vi "FTP自动升级更新main.vi"() -> ()   [LabVIEW 2016, in "自动更新.lvlib"]
uses:
  <vilib>/FTP/NI_FTP.lvlib
panel:
  out "有新版本":bool
  out "最新版本获取进度":u8(slide) scale=0.0..100.0
  # "版本获取中，请稍后！"
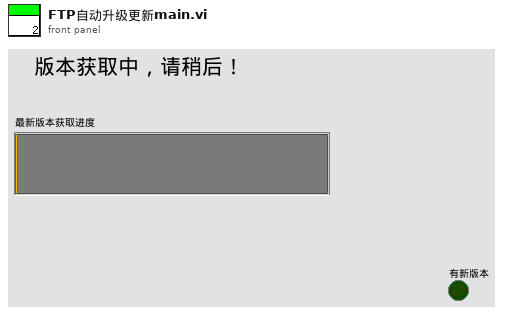
[diagram p1: front panel]
types:
  T1 = enum16{"get version information", "get success", "contact", "over"}
  T2 = cluster{"网络灯":bool, "接收中":bool, "已接收百分比":u8, "接收成功次数":dbl, "当前步骤":enum16{"init", "receivehead", "receivecontent", "receivesuccess", "over"}, "文件名":string, "error out":errorcluster}
  T3 = enum16{"open", "replace", "create", "open or create", "replace or create", "replace or create with confirmation"}
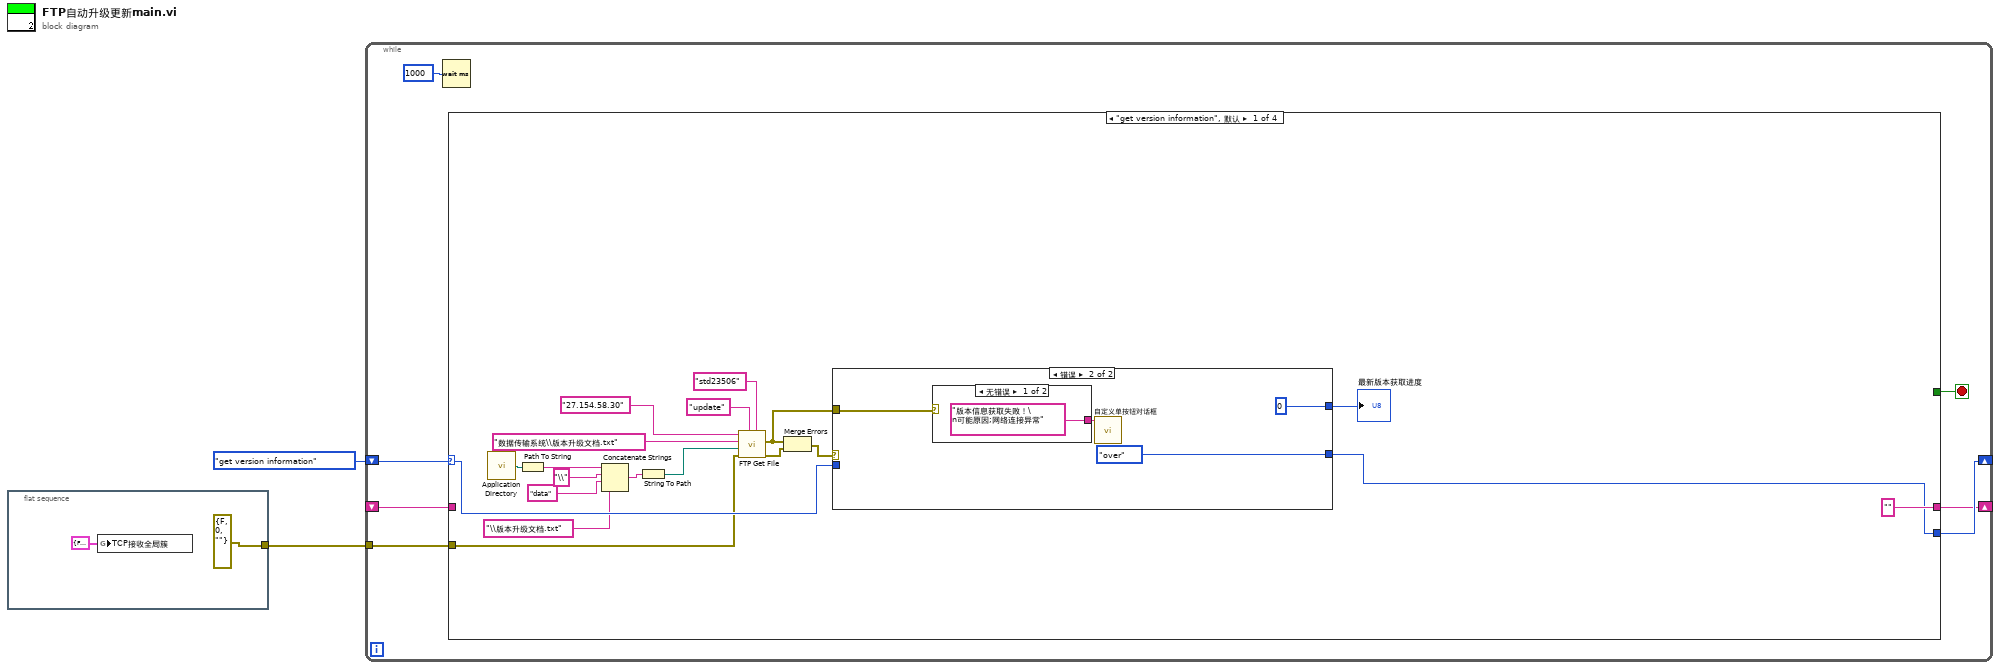
[diagram p0: block diagram]
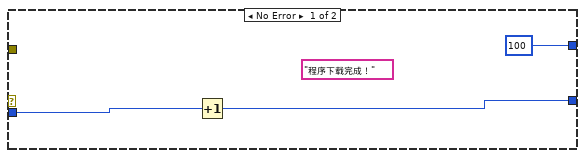
[diagram p2: hidden frame]
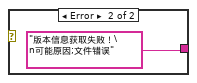
[diagram p3: hidden frame]
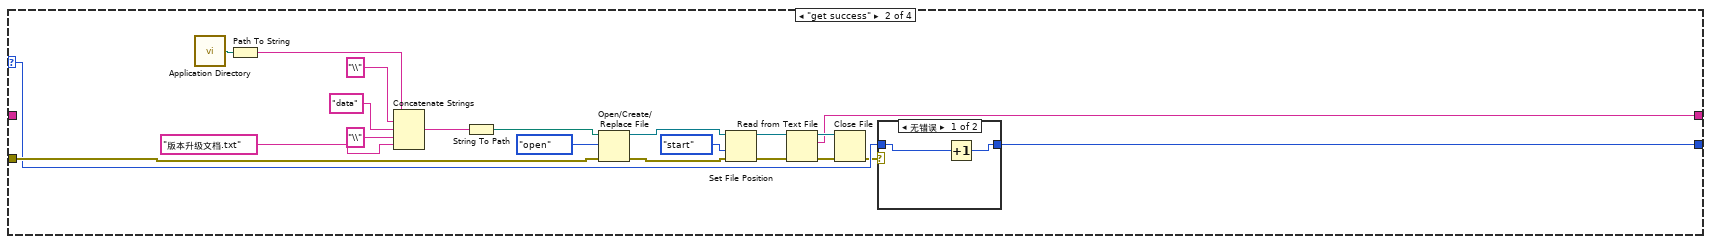
[diagram p4: hidden frame]
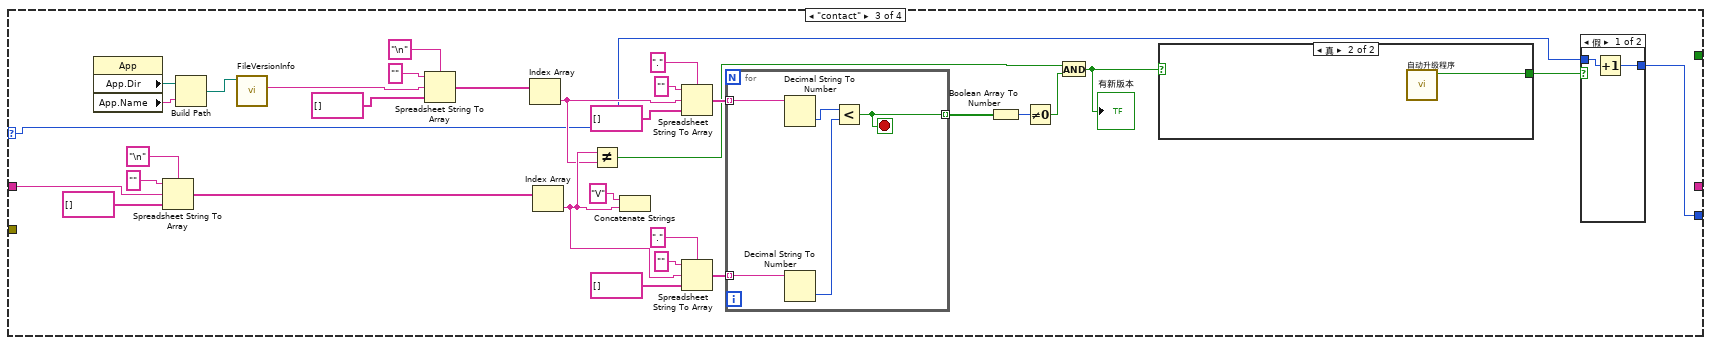
[diagram p6: hidden frame]
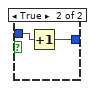
[diagram p7: hidden frame]
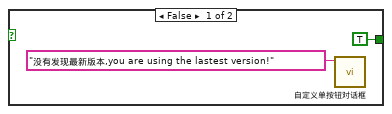
[diagram p8: hidden frame]
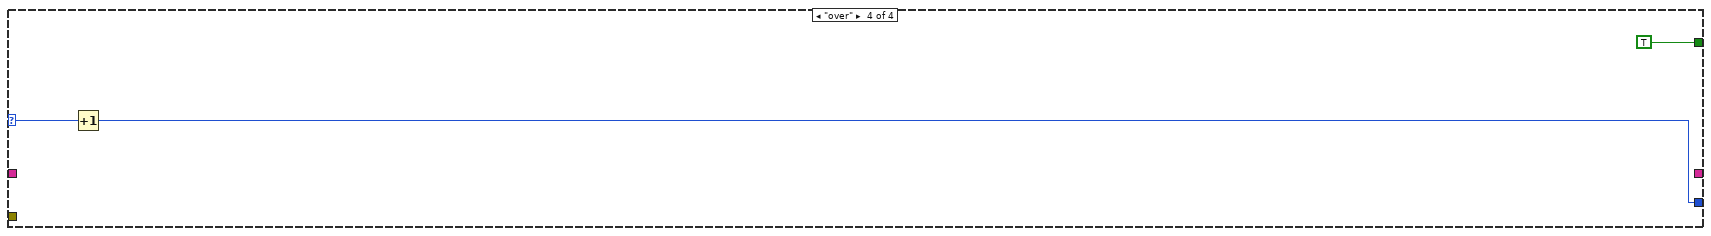
[diagram p9: hidden frame]
diagram:
  n1 = flat-sequence {
    tunnel: [errorcluster {"status"=FALSE, "code"=0, "source"=""} ("错误常量")] -> w1
    frame #0 {
      n2 = global write "全局变量1.vi" "TCP接收全局簇"(T2 {"网络灯"=FALSE, "接收中"=FALSE, "已接收百分比"=0, "接收成功次数"=0.0, "当前步骤"=enum."init", "文件名"="", "error out"={"status"=FALSE, "code"=0, "source"=""}} ("TCP接收全局簇")) -> ()
    }
  }
  n3 = while {
    shift-right: [w9] -> _
    shift-left: T1."get version information" -> [w10]
    tunnel: w1 -> [w8]
    shift-right: [w7] -> _
    shift-left: _ -> [w6]
    stop <- w5 stop-if-true
    n4 = Wait (ms)(milliseconds to wait=u32 1000 ("等待时间（毫秒）")) -> ()  [unwired: 1 out]
    n5 = case shown="\"get version information\", 默认" w10 {
      selector: w10 -> [w15 w47 w69 w109]
      tunnel: [w14 w46 w68 w108] -> w9
      tunnel: w8 -> [w13 w48 _ _]
      tunnel: ["" w40 _ _] -> w7
      tunnel: w6 -> [_ _ w72 _]
      tunnel: [_ _ _ TRUE] -> w5
      frame "get version information", Default {
        n6 = call <vilib>:"Application Directory.vi"() -> ("Application Directory"=w24:path)
        n7 = Path To String(path=w24) -> (string=w27:string)
        n8 = Concatenate Strings(w27, "\\" ("字符串"), "data" ("字符串"), "\\版本升级文档.txt") -> (w23:string)
        n9 = String To Path(string=w23) -> (path=w22:path)
        n10 = call <vilib>:"FTP Get File.vi"("password"="std23506", "user"="update", "error in (no error)"=w13, "local path"=w22, "remote path"="数据传输系统\\版本升级文档.txt", "host"="27.154.58.30") -> ("error out"=w19:errorcluster, "file error"=w17:errorcluster)  [unwired: 4 in]
        n11 = Merge Errors(w17, w19) -> (w18:errorcluster)
        n12 = case shown="错误" w18 {
          tunnel: w17 -> [_ w36]
          tunnel: [u8 100 ("y") u8 0 ("y")] -> w16
          tunnel: [w32 T1."over"] -> w14
          tunnel: w15 -> [w31 _]
          frame No Error {
            (unwired) "程序下载完成！"
            n13 = Increment(x=w31) -> (x+1=w32:T1)
          }
          frame Error {
            n14 = case shown="无错误" w36 {
              tunnel: ["版本信息获取失败！\n可能原因;网络连接异常" "版本信息获取失败！\n可能原因;文件错误"] -> w37
              frame No Error {
              }
              frame Error {
              }
            }
            n15 = call "自定义单按钮对话框.vi"("消息"=w37) -> ()  [unwired: 11 in]
          }
        }
        "最新版本获取进度" <- w16
      }
      frame "get success" {
        n16 = call <vilib>:"Application Directory.vi"() -> ("Application Directory"=w53:path)
        n17 = Path To String(path=w53) -> (string=w56:string)
        n18 = Concatenate Strings(w56, "\\" ("字符串"), "data" ("字符串"), "\\" ("字符串"), "版本升级文档.txt" ("字符串")) -> (w50:string)
        n19 = String To Path(string=w50) -> (path=w49:path)
        n20 = Open/Create/Replace File(file path (use dialog)=w49, error in=w48, operation (0:open)=T3."open" ("操作(0:open)")) -> (refnum out=w59:refnum<file>, error out=w58:errorcluster)  [unwired: 3 in, 1 out]
        n21 = Set File Position(refnum=w59, from (0:start)=enum16{"start", "end", "current"}."start" ("自（0:起始）"), error in=w58) -> (refnum out=w44:refnum<file>, error out=w43:errorcluster)  [unwired: 1 in]
        n22 = Read from Text File(file (use dialog)=w44, error in=w43) -> (refnum out=w45:refnum<file>, text=w40:string, error out=w42:errorcluster)  [unwired: 2 in, 1 out]
        n23 = Close File(refnum=w45, error in=w42) -> (error out=w41:errorcluster)  [unwired: 1 out]
        n24 = case shown="无错误" w41 {
          tunnel: w47 -> [w62 w63]
          tunnel: [w61 w63] -> w46
          frame No Error {
            n25 = Increment(x=w62) -> (x+1=w61:T1)
          }
          frame Error {
          }
        }
      }
      frame "contact" {
        n26 = property class="App"() -> ("App.Dir"=w66:path, "App.Name"=w67:string)  [unwired: 2 in, 2 out]
        n27 = Spreadsheet String To Array(delimiter (Tab)="\n" ("分隔符(Tab)"), format string="" ("格式字符串"), spreadsheet string=w72, array type (2D Dbl)=string[] []) -> (array=w91:string[])
        n28 = Build Path(base path=w66, name or relative path=w67) -> (appended path=w65:path)
        n29 = call <vilib>:"FileVersionInfo.vi"("Application Path in"=w65) -> ("File Version Info"=w64:string)  [unwired: 7 in, 3 out]
        n30 = Spreadsheet String To Array(delimiter (Tab)="\n" ("分隔符(Tab)"), format string="" ("格式字符串"), spreadsheet string=w64, array type (2D Dbl)=string[] []) -> (array=w84:string[])
        n31 = Index Array(array=w84) -> (element=w75:string)  [unwired: 1 in]
        n32 = Index Array(array=w91) -> (element=w76:string)  [unwired: 1 in]
        n33 = Not Equal?(x=w76, y=w75) -> (x != y?=w73:bool)
        n34 = Concatenate Strings("V" ("字符串"), w76) -> ()  [unwired: 1 out]
        n35 = Spreadsheet String To Array(delimiter (Tab)="." ("分隔符(Tab)"), format string="" ("格式字符串"), spreadsheet string=w75, array type (2D Dbl)=string[] []) -> (array=w79:string[])
        n36 = Spreadsheet String To Array(delimiter (Tab)="." ("分隔符(Tab)"), format string="" ("格式字符串"), spreadsheet string=w76, array type (2D Dbl)=string[] []) -> (array=w80:string[])
        n37 = for {
          tunnel: w80 -> [w105] mode=indexing
          tunnel: w79 -> [w107] mode=indexing
          tunnel: [w106] -> w78 mode=indexing
          stop <- w106 stop-if-true
          n38 = Decimal String To Number(string=w107) -> (number=w104:i32)  [unwired: 2 in, 1 out]
          n39 = Decimal String To Number(string=w105) -> (number=w103:i32)  [unwired: 2 in, 1 out]
          n40 = Less?(x=w104, y=w103) -> (x < y?=w106:bool)
        }
        n41 = Boolean Array To Number(Boolean array=w78) -> (number=w77:u32)
        n42 = Not Equal To 0?(x=w77) -> (x != 0?=w74:bool)
        n43 = And(x=w73, y=w74) -> (x .and. y?=w71:bool)
        "有新版本" <- w71
        n44 = case shown="真" w71 {
          tunnel: [TRUE ("确定") w102] -> w70
          frame False {
            n45 = call "自定义单按钮对话框.vi"("消息"="没有发现最新版本,you are using the lastest version!") -> ()  [unwired: 11 in]
          }
          frame True {
            n46 = call "自动升级程序.vi"() -> ("确定"=w102:bool)  [unwired: 10 in, 1 out]
          }
        }
        n47 = case shown="假" w70 {
          tunnel: w69 -> [w97 w99]
          tunnel: [w96 w98] -> w68
          frame False {
            n48 = Increment(x=w97) -> (x+1=w96:T1)
          }
          frame True {
            n49 = Increment(x=w99) -> (x+1=w98:T1)
          }
        }
      }
      frame "over" {
        n50 = Increment(x=w109) -> (x+1=w108:T1)
      }
    }
  }
